vi "GetMessageError.vi"(8 "error in (no error)":errorcluster, 11 "message in":T1) -> (0 "error out":errorcluster, 1 "error info":string, 2 "error code":i32, 3 "message out":T1, 5 "error name":string)   [LabVIEW 2017]
doc: "Returns any error information included in a message by the process that sent the message."
uses:
  <vilib>/addons/InsightCM/MessageBus/Base/controls/Message.ctl
  <vilib>/addons/InsightCM/MessageBus/Base/controls/MessageHeader.ctl
  <vilib>/addons/InsightCM/MessageBus/Base/controls/KeyValuePair.ctl
  <vilib>/addons/InsightCM/Utilities/PropertyHelpers/PropertyHelpers.lvlib
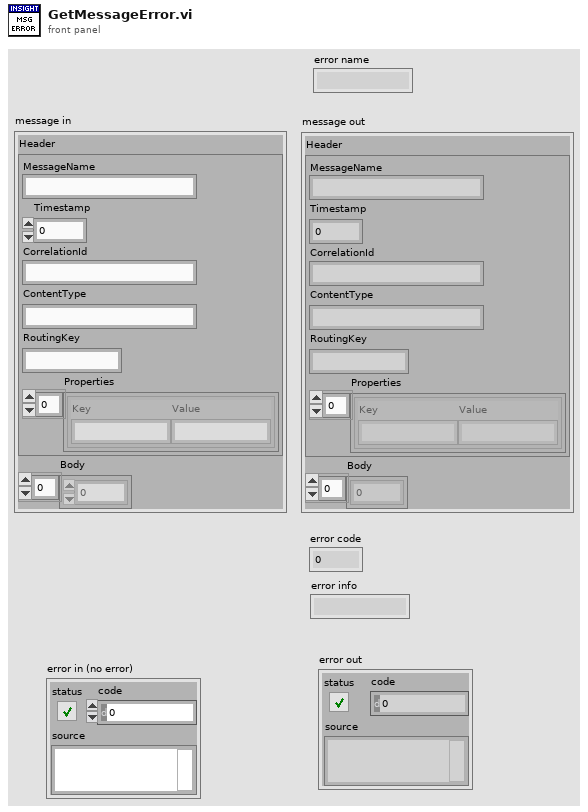
[diagram p1: front panel]
types:
  T1 = typedef "Message.ctl" = cluster{"Header":T2, "Body":u8[]}
  T2 = typedef "MessageHeader.ctl" = cluster{"MessageName":string, "Timestamp":i64, "CorrelationId":string, "ContentType":string, "RoutingKey":string, "Properties":T3[]}
  T3 = typedef "KeyValuePair.ctl" = cluster{"Key":string, "Value":string}
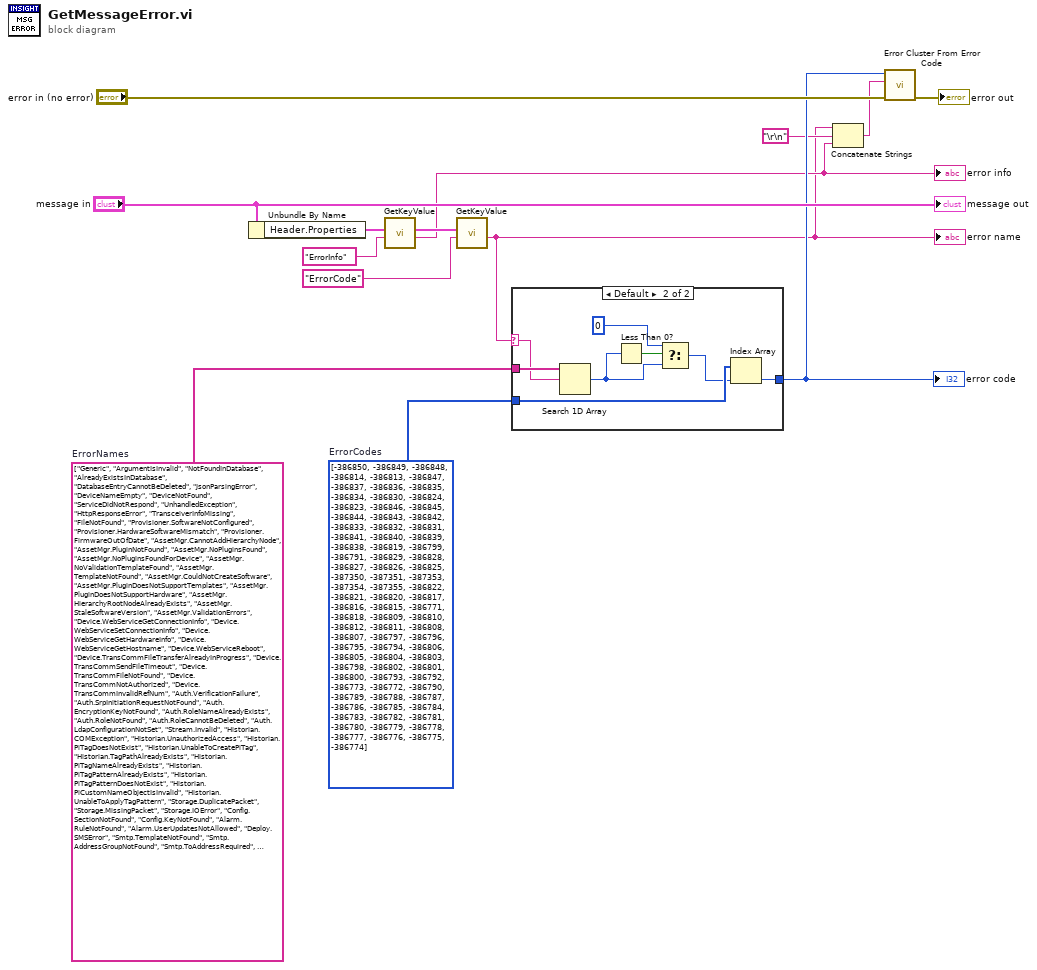
[diagram p0: block diagram]
diagram:
  w13 = i32[] [-386850, -386849, -386848, -386814, -386813, -386847, -386837, -386836, -386835, -386834, -386830, -386824, -386823, -386846, -386845, -386844, -386843, -386842, -386833, -386832, -386831, -386841, -386840, -386839, -386838, -386819, -386799, -386791, -386829, -386828, -386827, -386826, -386825, -387350, -387351, -387353, -387354, -387355, -386822, -386821, -386820, -386817, -386816, -386815, -386771, -386818, -386809, -386810, -386812, -386811, -386808, -386807, -386797, -386796, -386795, -386794, -386806, -386805, -386804, -386803, -386798, -386802, -386801, -386800, -386793, -386792, -386773, -386772, -386790, -386789, -386788, -386787, -386786, -386785, -386784, -386783, -386782, -386781, -386780, -386779, -386778, -386777, -386776, -386775, -386774]  # ErrorCodes
  w14 = string[] ["Generic", "ArgumentIsInvalid", "NotFoundInDatabase", "AlreadyExistsInDatabase", "DatabaseEntryCannotBeDeleted", "JsonParsingError", "DeviceNameEmpty", "DeviceNotFound", "ServiceDidNotRespond", "UnhandledException", "HttpResponseError", "TransceiverInfoMissing", "FileNotFound", "Provisioner.SoftwareNotConfigured", "Provisioner.HardwareSoftwareMismatch", "Provisioner.FirmwareOutOfDate", "AssetMgr.CannotAddHierarchyNode", "AssetMgr.PluginNotFound", "AssetMgr.NoPluginsFound", "AssetMgr.NoPluginsFoundForDevice", "AssetMgr.NoValidationTemplateFound", "AssetMgr.TemplateNotFound", "AssetMgr.CouldNotCreateSoftware", "AssetMgr.PluginDoesNotSupportTemplates", "AssetMgr.PluginDoesNotSupportHardware", "AssetMgr.HierarchyRootNodeAlreadyExists", "AssetMgr.StaleSoftwareVersion", "AssetMgr.ValidationErrors", "Device.WebServiceGetConnectionInfo", "Device.WebServiceSetConnectionInfo", "Device.WebServiceGetHardwareInfo", "Device.WebServiceGetHostname", "Device.WebServiceReboot", "Device.TransCommFileTransferAlreadyInProgress", "Device.TransCommSendFileTimeout", "Device.TransCommFileNotFound", "Device.TransCommNotAuthorized", "Device.TransCommInvalidRefNum", "Auth.VerificationFailure", "Auth.SrpInitiationRequestNotFound", "Auth.EncryptionKeyNotFound", "Auth.RoleNameAlreadyExists", "Auth.RoleNotFound", "Auth.RoleCannotBeDeleted", "Auth.LdapConfigurationNotSet", "Stream.Invalid", "Historian.COMException", "Historian.UnauthorizedAccess", "Historian.PiTagDoesNotExist", "Historian.UnableToCreatePiTag", "Historian.TagPathAlreadyExists", "Historian.PiTagNameAlreadyExists", "Historian.PiTagPatternAlreadyExists", "Historian.PiTagPatternDoesNotExist", "Historian.PiCustomNameObjectIsInvalid", "Historian.UnableToApplyTagPattern", "Storage.DuplicatePacket", "Storage.MissingPacket", "Storage.IOError", "Config.SectionNotFound", "Config.KeyNotFound", "Alarm.RuleNotFound", "Alarm.UserUpdatesNotAllowed", "Deploy.SMSError", "Smtp.TemplateNotFound", "Smtp.AddressGroupNotFound", "Smtp.ToAddressRequired", "Smtp.InvalidServiceConfiguration", "Analysis.StreamPrepError", "Analysis.NotStreamingBlockReceived", "Analysis.NotStreamingStreamStopReceived", "Analysis.UnpackJsonStateStringError", "Analysis.UnknownJsonStateStringMessageType", "Analysis.JsonStateMessageConversionError", "Analysis.FileOpenFailure", "Analysis.HierarchyPropsNotFound", "Analysis.ReferenceChannelNotFound", "Analysis.ReferenceTypeNotFound", "Analysis.SpeedPropertyNotFound", "Analysis.UnknownFeatureCodeName", "Analysis.UnitStringNotFound", "Analysis.UnitConversionUnsuccessful", "Analysis.InvalidAmplitudeScale", "Analysis.SpectralBandCacheError", "Analysis.UnknownInternalMessage"]  # ErrorNames
  n1 = Unbundle By Name("message in") -> ("Header.Properties"=w12:T3[])
  n2 = call <vilib>:"GetKeyValue.vi"("key"="ErrorInfo" ("Key"), "key value pairs"=w12) -> ("value"=w3:string, "key value pairs out"=w11:T3[])  [unwired: 7 in, 1 out]
  "error info" <- w3
  n3 = call <vilib>:"GetKeyValue.vi"("key"="ErrorCode" ("Key"), "key value pairs"=w11) -> ("value"=w2:string)  [unwired: 7 in, 2 out]
  "error name" <- w2
  n4 = case shown="Default" w2 {
    selector: w2 -> [_ w15]
    tunnel: w14 -> [_ w22]
    tunnel: w13 -> [_ w21]
    tunnel: [_ w20] -> w5
    frame "" {
    }
    frame Default {
      n5 = Search 1D Array(1D array=w22, element=w15) -> (index of element=w18:i32)  [unwired: 1 in]
      n6 = Less Than 0?(x=w18) -> (x < 0?=w19:bool)
      n7 = Select(t=0, s=w19, f=w18) -> (s? t:f=w17:i32)
      n8 = Index Array(array=w21, index=w17) -> (element=w20:i32)
    }
  }
  "error code" <- w5
  n9 = Concatenate Strings(w2, "\r\n", w3) -> (w1:string)
  n10 = call <vilib>:"Error Cluster From Error Code.vi"("error in (no error)"="error in (no error)", "error message (\"\")"=w1, "error code (0)"=w5) -> ("error out"=→"error out":errorcluster)  [unwired: 6 in]
  "message out" <- "message in"
